vi "Main.vi"() -> ()   [LabVIEW 2015]
doc: "The myRIO Project template acquires acceleration data from the onboard accelerometer and displays the changes of acceleration values in a waveform chart."
uses:
  <vilib>/vision/driver/IMAQdx.llb/IMAQdx Acquisition Mode.ctl
  <vilib>/vision/driver/IMAQdx.llb/IMAQdx Buffer Number Mode.ctl
  <vilib>/vision/driver/NI_Vision_Acquisition_Software.lvlib
  <vilib>/vision/NI_Vision_Development_Module.lvlib
panel:
  in  "Match Saturation Threshold (Color Matching 1)":i32=80
  out "Match Score (Color Matching 1)":i32[](array[numeric])
  out "Match Flag (Color Matching 1)":bool[](array[boolean])
  in  "Camera Name":refnum<k21> caption="IMAQdx Session"
  in  "Stop":bool
  out "Frame Rate":dbl(knob) scale=0.0..100.0
  out "Image":T1(plugin-control)
  out "Buffer Number":u32
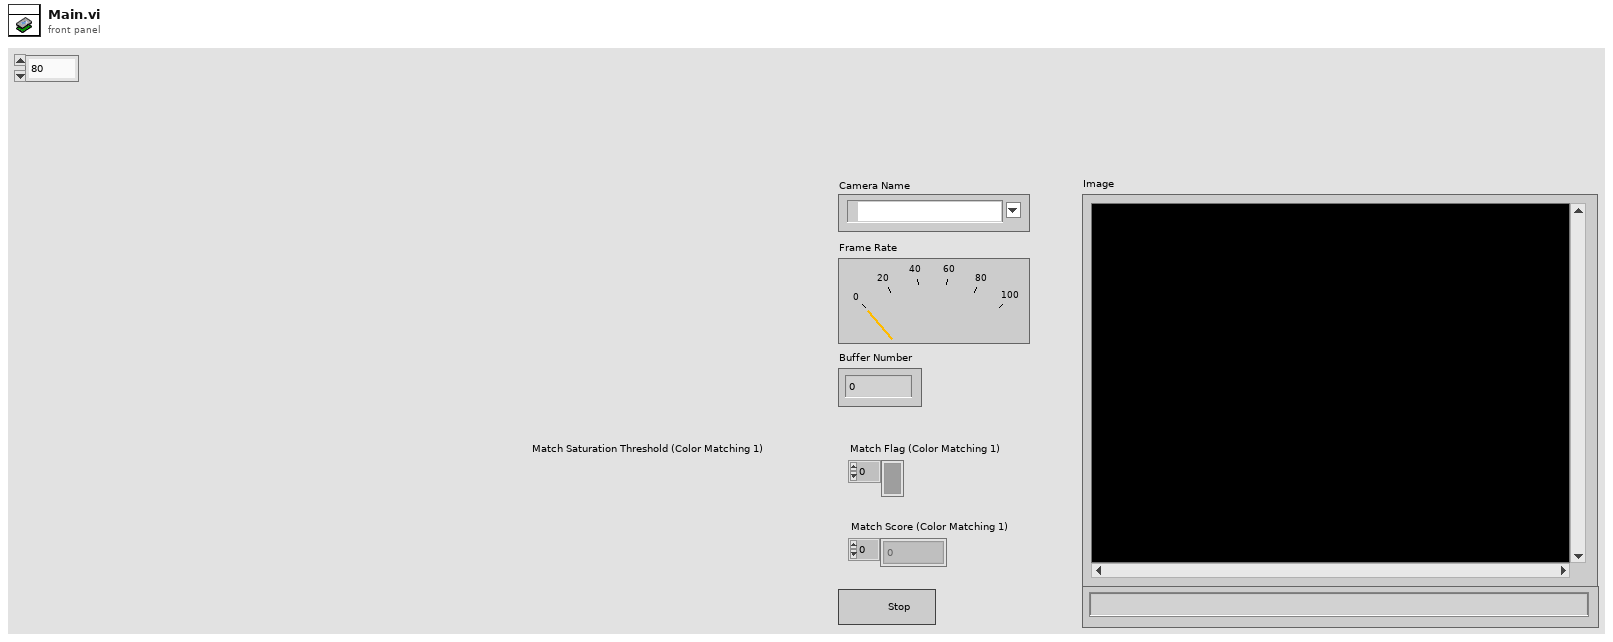
[diagram p1: front panel]
types:
  T1 = typedef "IMAQ Image.ctl" = refnum<image>
  T2 = typedef "NI_Vision_Acquisition_Software.lvlib/IMAQdx Acquisition Mode.ctl" = enum32{"One Shot", "Continuous"}
  T3 = typedef "IMAQdx.ctl" = refnum<k21>
  T4 = cluster{"Global Rectangle":i32[], "Contours":cluster{"ID":enum32{"External", "Internal"}, "Type":u32, "Coordinates":i32[]}[]}
  T5 = typedef "NI_Vision_Acquisition_Software.lvlib/IMAQdx Buffer Number Mode.ctl" = enum32{"Next", "Last", "Buffer Number", "Every", "Last New"}
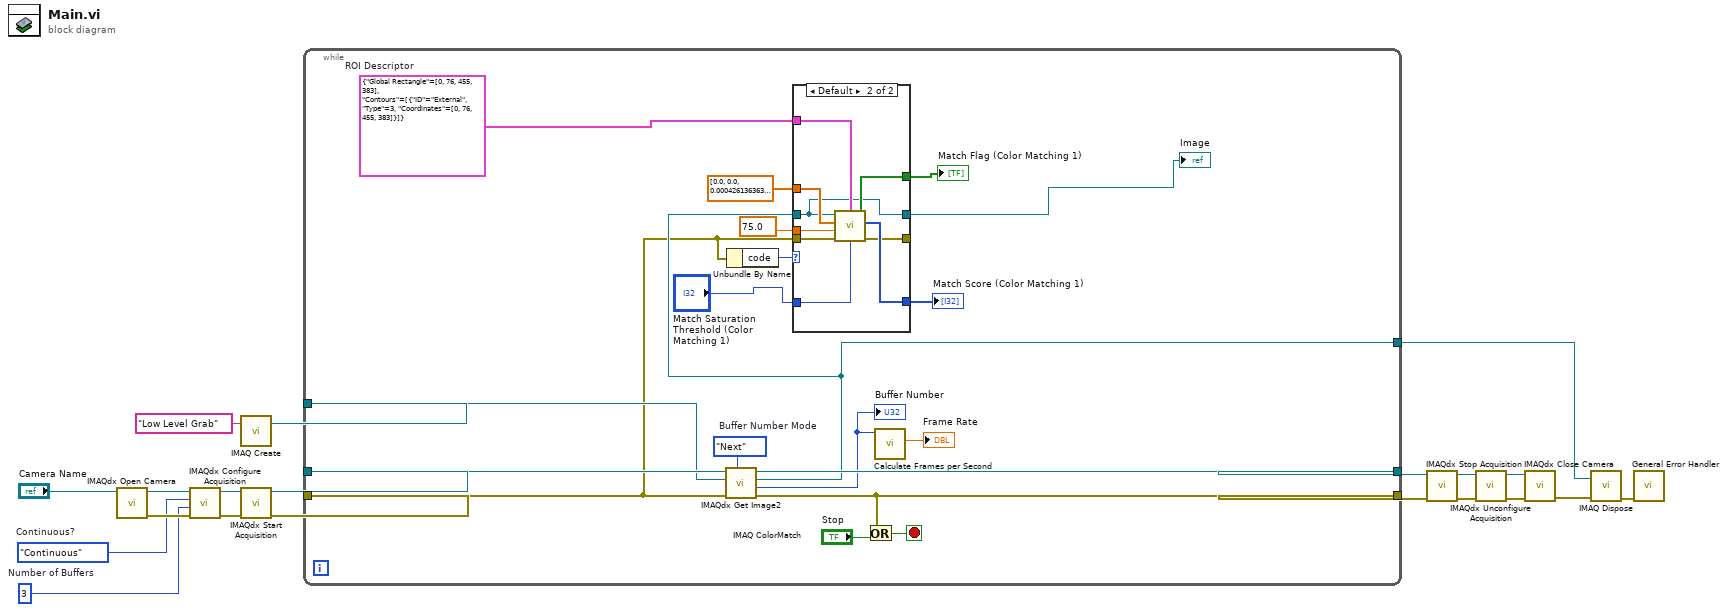
[diagram p0: block diagram]
diagram:
  w11 = u32 3  # Number of Buffers
  w12 = IMAQdx_Acquisition_Mode."Continuous"  # Continuous?
  n1 = call <vilib>:"IMAQdx Open Camera.vi"("Session In"="Camera Name") -> ("error out"=w15:errorcluster, "Session Out"=w18:T3)  [unwired: 2 in, 7 out]
  n2 = call <vilib>:"IMAQdx Configure Acquisition.vi"("error in"=w15, "Number of Buffers"=w11, "Continuous?"=w12, "Session In"=w18) -> ("error out"=w14:errorcluster, "Session Out"=w17:T3)  [unwired: 6 out]
  n3 = call "IMAQ Create"("Image Name"="Low Level Grab") -> ("New Image"=w20:T1)  [unwired: 3 in, 2 out]
  n4 = call <vilib>:"IMAQdx Start Acquisition.vi"("error in"=w14, "Session In"=w17) -> ("error out"=w13:errorcluster, "Session Out"=w16:T3)  [unwired: 8 out]
  n5 = while {
    tunnel: [w36] -> w9
    tunnel: w13 -> [w22]
    tunnel: w16 -> [w38]
    tunnel: [w32] -> w10
    tunnel: w20 -> [w37]
    tunnel: [w23] -> w1
    stop <- w39 stop-if-true
    w25 = T4 {"Global Rectangle"=[0, 76, 455, 383], "Contours"=[{"ID"=enum."External", "Type"=3, "Coordinates"=[0, 76, 455, 383]}]}  # ROI Descriptor
    w34 = IMAQdx_Buffer_Number_Mode."Next"  # Buffer Number Mode
    n6 = call <vilib>:"IMAQdx Get Image2.vi"("Buffer Number Mode (Next)"=w34, "error in"=w22, "Image In"=w37, "Session In"=w38) -> ("error out"=w32:errorcluster, "Buffer Number Out"=w33:u32, "Image Out"=w23:T1, "Session Out"=w36:T3)  [unwired: 4 in]
    "Buffer Number" <- w33
    n7 = Unbundle By Name(w22) -> ("code"=w24:i32)
    n8 = case shown="Default" w24 {
      tunnel: 75.0 ("Minimum Match Score") -> [_ w49]
      tunnel: "Match Saturation Threshold (Color Matching 1)" -> [_ w48]
      tunnel: dbl[] [0.0, 0.0, 0.0004261363636363636, 0.0, 0.007244318181818182, 0.020170454545454547, 0.06491477272727272, 0.9058238636363637, 0.00014204545454545454, 0.0, 0.0, 0.0, 0.0, 0.0, 0.0, 0.001278409090909091] ("Color Spectrum") -> [_ w47]
      tunnel: [_ w46] -> w27
      tunnel: [_ w45] -> w26
      tunnel: w23 -> [w40 w41]
      tunnel: w22 -> [_ w44]
      tunnel: [_ w43] -> _
      tunnel: w25 -> [_ w42]
      tunnel: [w40 w41] -> w21
      frame -1074396199, -1074396198 {
        # "Discard\nCoordinate\nSystem Error"
      }
      frame Default {
        n9 = call "IMAQ ColorMatch"("ROI Descriptor"=w42, "Image"=w41, "Color Spectrum"=w47, "Match Saturation Threshold"=w48, "Minimum Match Score"=w49, "error in (no error)"=w44) -> ("Match Flag"=w46:bool[], "Match Score"=w45:i32[], "error out"=w43:errorcluster)  [unwired: 1 out]
      }
    }
    "Image" <- w21
    "Match Flag (Color Matching 1)" <- w27
    "Match Score (Color Matching 1)" <- w26
    n10 = Or(x=w32, y="Stop") -> (x .or. y?=w39:bool)
    n11 = call <vilib>:"Calculate Frames per Second.vi"("Buffer Number"=w33) -> ("Processed Frames/s"=→"Frame Rate":dbl)  [unwired: 8 in, 2 out]
  }
  n12 = call <vilib>:"IMAQdx Stop Acquisition.vi"("error in"=w10, "Session In"=w9) -> ("error out"=w5:errorcluster, "Session Out"=w6:T3)  [unwired: 8 out]
  n13 = call <vilib>:"IMAQdx Unconfigure Acquisition.vi"("error in"=w5, "Session In"=w6) -> ("error out"=w8:errorcluster, "Session Out"=w7:T3)  [unwired: 8 out]
  n14 = call <vilib>:"IMAQdx Close Camera.vi"("error in"=w8, "Session In"=w7) -> ("error out"=w4:errorcluster)  [unwired: 9 out]
  n15 = call "IMAQ Dispose"("Image"=w1, "error in (no error)"=w4) -> ("error out"=w3:errorcluster)  [unwired: 4 in]
  n16 = call <vilib>:"General Error Handler.vi"("error in (no error)"=w3) -> ()  [unwired: 2 in, 13 out]
